vi "CCP_Main.vi"() -> ()   [LabVIEW 2019]
uses:
  LabJackU3/temperature_status_LabJackU3.ctl
panel:
  in  "open_IVC_OC200":bool caption="open_THCD_400"
  out "IVC_OC200_P2":dbl caption="IVC P2" format="%_3e"
  out "IVC_OC200_P1":dbl caption="IVC P1" format="%_3e"
  out "IVC_OC200_ST":u32(colorbox)
  out "HeatTape_ST":u32(colorbox)
  in  "open_Heat_Tape":bool caption="open_THCD_400"
  in  "audio_onoff":bool caption="Audio Alarm"
  in  "disp_magnet_level":bool
  in  "disp_shell_volume":bool
  in  "disp_magnet_space":bool
  out "MccHat_P":dbl caption="psig" format="%.2f"
  out "MccHat_ST":u32(colorbox)
  in  "open_MccHat":bool caption="open_THCD_400"
  out "LJT4_P_HR3":dbl caption="psi" format="%.1f"
  out "FM2":dbl
  out "msg_subsys":string
  in  "open_LJT4":bool caption="open_THCD_400"
  out "LJT4_T":dbl caption="°F" format="%.1f"
  out "LJT4_P":dbl caption="psi" format="%.1f"
  out "LJT4_ST":u32(colorbox)
  in  "open_GVB":bool caption="open_THCD_400"
  out "GVB_turn":dbl caption="turn" format="%.2f"
  out "GVB_ST":u32(colorbox)
  out "MRB_opening":dbl caption="%"
  in  "open_MRB":bool caption="open_THCD_400"
  out "MRB_ST":u32(colorbox)
  in  "Interval":i32=1000 caption="ms"
  out "time_update":timestamp caption="Last Update" format="%<%Y-%m-%d %H:%M:%S>T"
  out "MagPS_ST":u32(colorbox)
  out "ITM10_ST":u32(colorbox)
  out "RPLCW_ST":u32(colorbox)
  out "LJU3_TC_ST":u32(colorbox)
  out "LS218_02_ST":u32(colorbox)
  out "LS218_01_ST":u32(colorbox)
  out "MCCETC03_T7":dbl caption="F" format="%.1f"
  out "MCCETC03_T6":dbl caption="F" format="%.1f"
  out "MCCETC03_ST":u32(colorbox)
  out "MCCETC02_ST":u32(colorbox)
  out "MCCETC01_ST":u32(colorbox)
  out "TPG361_ST":u32(colorbox)
  out "BGA244_ST":u32(colorbox)
  out "THCD401_ST":u32(colorbox)
  out "MG_ST":u32(colorbox)
  out "FV_ST":u32(colorbox)
  out "MKS670_He3_ST":u32(colorbox)
  out "MKS670_100_ST":u32(colorbox)
  out "MKS670_1000_ST":u32(colorbox)
  in  "control_lock":bool caption="Control"
  in  "stop_all":bool caption="open_THCD_400"
  in  "start_all":bool caption="open_THCD_400"
  out "MKS946_ST":u32(colorbox)
  out "LS218_02_T8":dbl format="%.1f"
  out "level_fridge_LHe":dbl(slide) caption="%" scale=0.0..45.0 scale format="%#.1f"
  out "level_fridge_LN2":dbl(slide) caption="%" scale=0.0..100.0 scale format="%#.1f"
  out "MCCETC02_T7":dbl caption="Sep. Line" format="%.1f"
  in  "open_RPLCW":bool caption="open_THCD_400"
  out "RPLCW_WFS1":dbl caption="WFS1" format="%.1f"
  out "RPLCW_M4":dbl caption="M4" format="%.1f"
  out "RPLCW_M3":dbl caption="M3" format="%.1f"
  out "PRLCW_M2":dbl caption="M2" format="%.1f"
  out "RPLCW_M1":dbl caption="M1" format="%.1f"
  in  "open_LS218_02":bool caption="open_THCD_400"
  out "LS218_02_T7":dbl format="%.1f"
  out "LS218_02_T6":dbl format="%.1f"
  out "LS218_02_T5":dbl format="%.1f"
  out "LS218_02_T4":dbl format="%.1f"
  out "LS218_02_T3":dbl caption="W" format="%.1f"
  out "LS218_02_T2":dbl format="%.1f"
  out "LS218_02_T1":dbl caption="W" format="%.1f"
  out "Nose LHe Level":dbl(slide) caption="%" scale=0.0..100.0 scale format="%#_1f"
  in  "open_MagPS":bool caption="open_THCD_400"
  out "LS218_01_T8":dbl caption="W"
  out "LS218_01_T7":dbl caption="W"
  out "LS218_01_T6":dbl caption="W"
  out "LS218_01_T5":dbl caption="W"
  out "LS218_01_T4":dbl caption="W"
  out "LS218_01_T3":dbl caption="W"
  out "LS218_01_T2":dbl caption="W"
  out "LS218_01_T1":dbl caption="W"
  out "FC1":dbl
  out "FC2":dbl
  out "FM1":dbl
  in  "open_THCD_401":bool caption="open_THCD_400"
  out "MCCETC03_T5":dbl format="%.1f"
  out "MCCETC03_T4":dbl format="%.1f"
  in  "open_ITM10":bool caption="open_THCD_400"
  out "T_Coil_B":dbl caption="Coil B"
  out "T_Coil_T":dbl caption="Coil T"
  out "T_Tank_B":dbl caption="Tank B"
  out "T_Tank_T":dbl caption="Tank T"
  out "MG5":dbl caption="psi" format="%.1f"
  in  "open_LJU3_TC":bool caption="open_THCD_400"
  out "LJU3_T_status":T1=enum."UNKNOWN" caption="QT Comp. LCW Temp."
  out "p_mks670_100":dbl caption="Torr"
  in  "open_LS218_01":bool caption="open_THCD_400"
  in  "open_MCCETC03":bool caption="open_THCD_400"
  out "MCCETC03_T3":dbl caption="T3" format="%.1f"
  out "MCCETC03_T2":dbl caption="T2" format="%.1f"
  out "MCCETC03_T1":dbl caption="T1" format="%.1f"
  out "MCCETC03_T0":dbl caption="T0" format="%.1f"
  in  "open_MCCETC01":bool caption="open_THCD_400"
  out "MCCETC01_T7":dbl caption="DR" format="%.1f"
  out "MCCETC01_T6":dbl caption="DL" format="%.1f"
  out "MCCETC01_T5":dbl caption="DB" format="%.1f"
  out "MCCETC01_T4":dbl caption="DT" format="%.1f"
  out "MCCETC01_T3":dbl caption="UR" format="%.1f"
  out "MCCETC01_T2":dbl caption="UL" format="%.1f"
  out "MCCETC01_T1":dbl caption="UB" format="%.1f"
  out "MCCETC01_T0":dbl caption="UT" format="%.1f"
  out "MCCETC02_T6":dbl caption="Sep. Line" format="%.1f"
  out "MCCETC02_T5":dbl caption="LHe FL #2" format="%.1f"
  out "MCCETC02_T4":dbl caption="LHe FL #1" format="%.1f"
  out "MCCETC02_T3":dbl caption="LHe FL Stinger" format="%.1f"
  out "MCCETC02_T2":dbl caption="Fridge Top" format="%.1f"
  in  "open_MCCETC02":bool caption="open_THCD_400"
  out "MCCETC02_T1":dbl caption="IVC Top" format="%.2f"
  out "MCCETC02_T0":dbl caption="IVC Bottom" format="%.2f"
  in  "open_TPG361":bool caption="open_THCD_400"
  out "TPG361_p":dbl caption="IVC" format="%_3e"
  in  "open_BGA244":bool caption="open_THCD_400"
  out "Purity":dbl caption="%" format="%.2f"
  in  "stop":bool
  in  "open_MaxiGauge":bool
  out "MG4":dbl format="%_4f"
  out "MG3":dbl format="%_4f"
  out "MG2":dbl caption="Torr" format="%_4f"
  out "MG1":dbl caption="Torr" format="%_4f"
  in  "open_Fridge_Valve":bool
  in  "open_MKS670_He3":bool
  in  "open_MKS670_100":bool
  in  "open_MKS670_1000":bool
  out "Bypass Valve":dbl format="%_3f"
  out "P2":dbl caption="Root Exhaust" format="%.2f"
  out "He3 Vapor Pressure":dbl
  out "p_mks670_1000":dbl caption="Torr"
  out "Run-Valve":dbl format="%_3f"
  out "P1":dbl caption="QT Manifold" format="%.2f"
  in  "open_MKS946":bool
  # "Expert Control"
  # "Cryo Control Panel"
  # "Fridge Temperatures"
  # "GPM"
  # "Torr"
  # "Click a reading and stay for 1 sec to find its controller name."
  # "psi"
  # "Controller"
  # "Status"
  # "Sub Panel"
  # "MKS 670 / 1000"
  # "Fridge pressure upto 1000 Torr."
  # "Microwave System"
  # "L/m"
  # "EIO Tube"
  # "EIO Top"
  # "MKS 670 /   100"
  # "Fridge pressure upto 100 Torr."
  # "psi"
  # "°C"
  # "MKS 670 / He3"
  # "Fridge pressure with He3 probe."
  # "MKS 946"
  # "Return line pressures."
  # "THCD-401"
  # "Return flow control/monitor."
  # "Turns"
  # "MaxiGauge"
  # "Return line pressures."
  # "L/m"
  # "L/m"
  # "Outside gHe Tank"
  # "°C"
  # "°C"
  # "Fridge Valve"
  # "Fridge valves.  LHe level."
  # "Auto"
  # "Torr"
  # "Torr"
  # "BGA244"
  # "Helium purity."
  # "°C"
  # "HR3"
  # "TPG361"
  # "IVC pressure."
  # "L/m"
  # "ITM10"
  # "Magnet temperatures."
  # "Turns"
  # "MCC E-TC #01"
  # "Magnet pipe temperatures."
  # "MCC E-TC #02"
  # "Surface temperatures."
  # "K"
  # "MCC E-TC #03"
  # "Annealing, microwave, and heat-tape temp."
  # "°C"
  # "K"
  # "Target-Cup\nTemperatures"
  # "LakeShore218 #01"
  # "Fridge temperatures."
  # "°C"
  # "°C"
  # "LakeShore218 #02"
  # "Target temperatures."
  # "Roots-Pump LCW"
  # "Roots-pump LCW flows."
  # "K"
  # "°C"
  # "K"
  # "LabJack U3"
  # "Compressor LCW temperatures."
  # "Torr"
  # "LabJack T4"
  # "Outside gHe tank."
  # "K"
  # "Magnet PS"
  # "Magnet current.  LHe & LN2 levels."
  # "W"
  # "°C"
  # "%"
  # "MR Bypass"
  # "Magnet return bypass valve."
  # "Auto"
  # "K"
  # "GV Bypass"
  # "Gate-valve bypass valve."
  # "Auto"
  # "K"
  # "MCC HAT #01"
  # "Magnet pressure."
  # "Magnet Surface Temperature"
  # "%"
  # "°C"
  # "Heat Tape"
  # "IVC & Turret heat tape."
  # "K"
  # "IVC Turbo Pressure"
  # "IVC_OC200"
  # "Schematic Version 8.0"
  # "K"
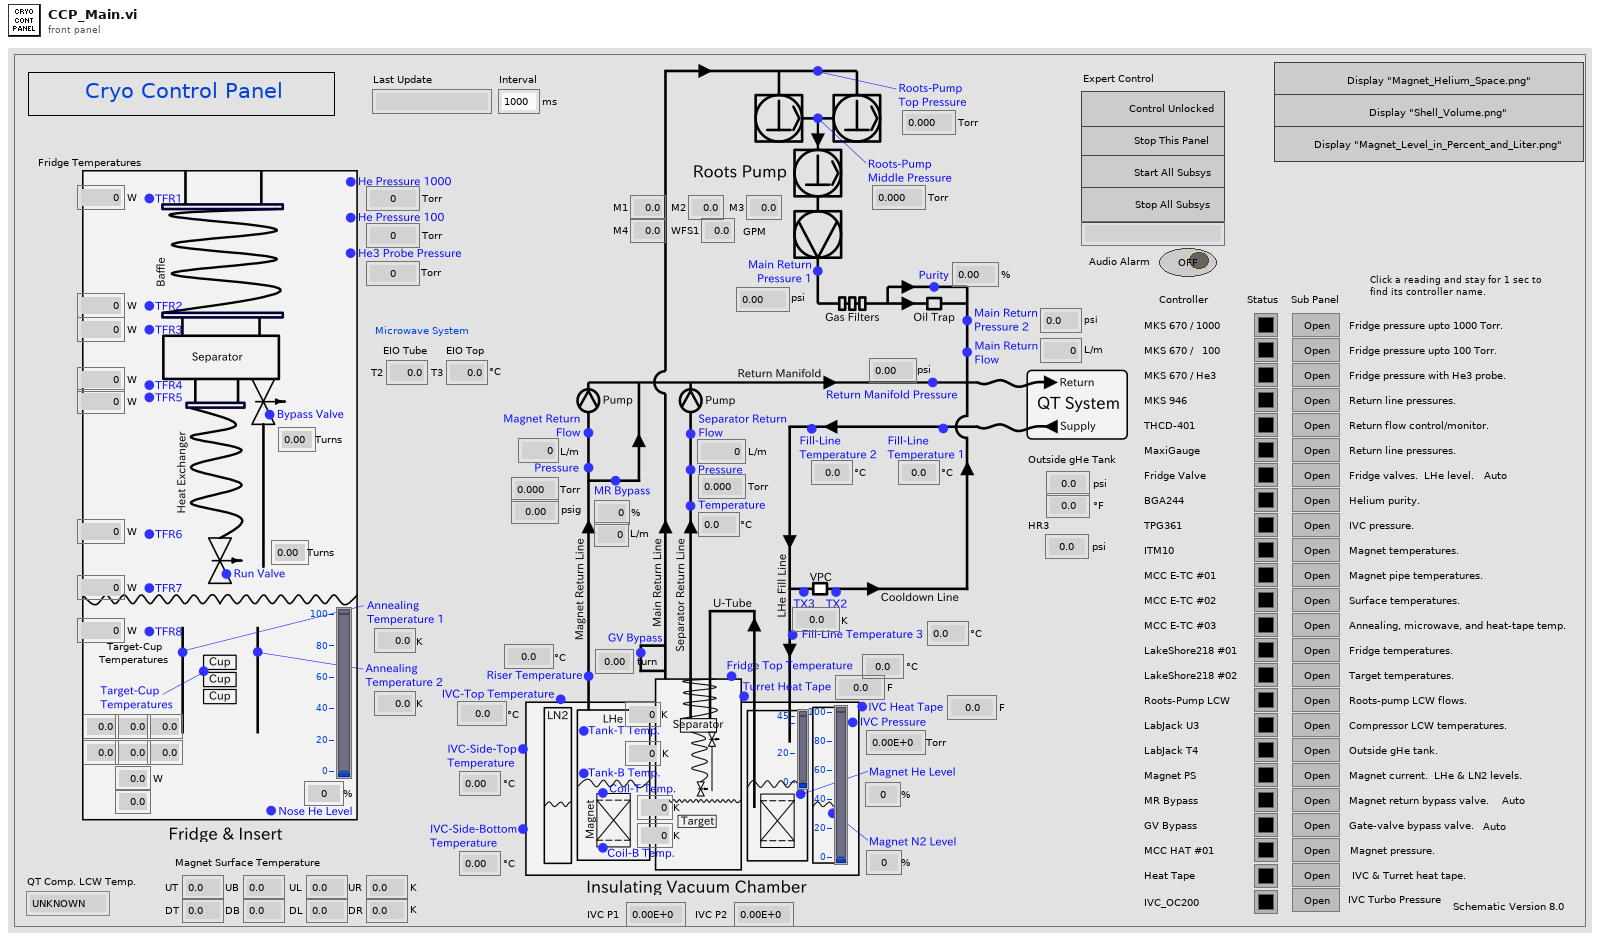
[diagram p1: front panel]
types:
  T1 = typedef "temperature_status_LabJackU3.ctl" = enum16{"OK", "UNKNOWN", "WARNING", "ERROR"}
  T2 = enum8{"Enabled", "Disabled", "Disabled and Grayed Out"}
  T3 = enum32{"Bad", "Idle", "Run top level", "Running"}
  T4 = cluster{"ITM10_ST":u32, "ITM10_Tank_T":dbl, "ITM10_Tank_B":dbl, "ITM10_Coil_T":dbl, "ITM10_Coil_B":dbl}
  T5 = cluster{"THCD401_ST":u32, "THCD401_FC1":dbl, "THCD401_FC2":dbl, "THCD401_FM1":dbl, "THCD401_FM2":dbl}
  T6 = cluster{"FV_ST":u32, "FV_run_valve":dbl, "FV_bypass_valve":dbl, "FV_nose_level":dbl}
  T7 = cluster{"MG_ST":u32, "MG_P1":dbl, "MG_P2":dbl, "MG_P3":dbl, "MG_P4":dbl, "MG_P5":dbl}
  T8 = cluster{"MKS670_1000_ST":u32, "MKS670_1000_P":dbl, "MKS670_1000_ST":u32, "MKS670_100_P":dbl, "MKS670_1000_ST":u32, "MKS670_He3_P":dbl}
  T9 = cluster{"MKS670_1000_ST":u32, "MKS946_P1":dbl, "MKS946_P2":dbl}
  T10 = cluster{"RPLCW_ST":u32, "RPLCW_M1":dbl, "RPLCW_M2":dbl, "RPLCW_M3":dbl, "RPLCW_M4":dbl, "RPLCW_WFS1":dbl}
  T11 = cluster{"LS218_02_ST":u32, "LS218_02_T1":dbl, "LS218_02_T2":dbl, "LS218_02_T3":dbl, "LS218_02_T4":dbl, "LS218_02_T5":dbl, "LS218_02_T6":dbl, "LS218_02_T7":dbl, "LS218_02_T8":dbl}
  T12 = cluster{"LS218_01_ST":u32, "LS218_01_T1":dbl, "LS218_01_T2":dbl, "LS218_01_T3":dbl, "LS218_01_T4":dbl, "LS218_01_T5":dbl, "LS218_01_T6":dbl, "LS218_01_T7":dbl, "LS218_01_T8":dbl}
  T13 = cluster{"MCCETC03_ST":u32, "MCCETC03_T0":dbl, "MCCETC03_T1":dbl, "MCCETC03_T2":dbl, "MCCETC03_T3":dbl, "MCCETC03_T4":dbl, "MCCETC03_T5":dbl, "MCCETC03_T6":dbl, "MCCETC03_T7":dbl}
  T14 = cluster{"MCCETC02_ST":u32, "MCCETC02_T0":dbl, "MCCETC02_T1":dbl, "MCCETC02_T2":dbl, "MCCETC02_T3":dbl, "MCCETC02_T4":dbl, "MCCETC02_T5":dbl, "MCCETC02_T6":dbl, "MCCETC02_T7":dbl}
  T15 = cluster{"MCCETC01_ST":u32, "MCCETC01_T0":dbl, "MCCETC01_T1":dbl, "MCCETC01_T2":dbl, "MCCETC01_T3":dbl, "MCCETC01_T4":dbl, "MCCETC01_T5":dbl, "MCCETC01_T6":dbl, "MCCETC01_T7":dbl}
  T16 = cluster{"LJT4_ST":u32, "LJT4_P":dbl, "LJT4_T":dbl, "LJT4_P_HR3":dbl}
  T17 = cluster{"MagPS_ST":u32, "MagPS_LHe":dbl, "MagPS_LN2":dbl}
  T18 = cluster{"HeatTape_ST":u32, "HeatTape_T1":dbl, "HeatTape_T2":dbl}
  T19 = cluster{"IVC_OC200_ST":u32, "IVC_OC200_P1":dbl, "IVC_OC200_P2":dbl}
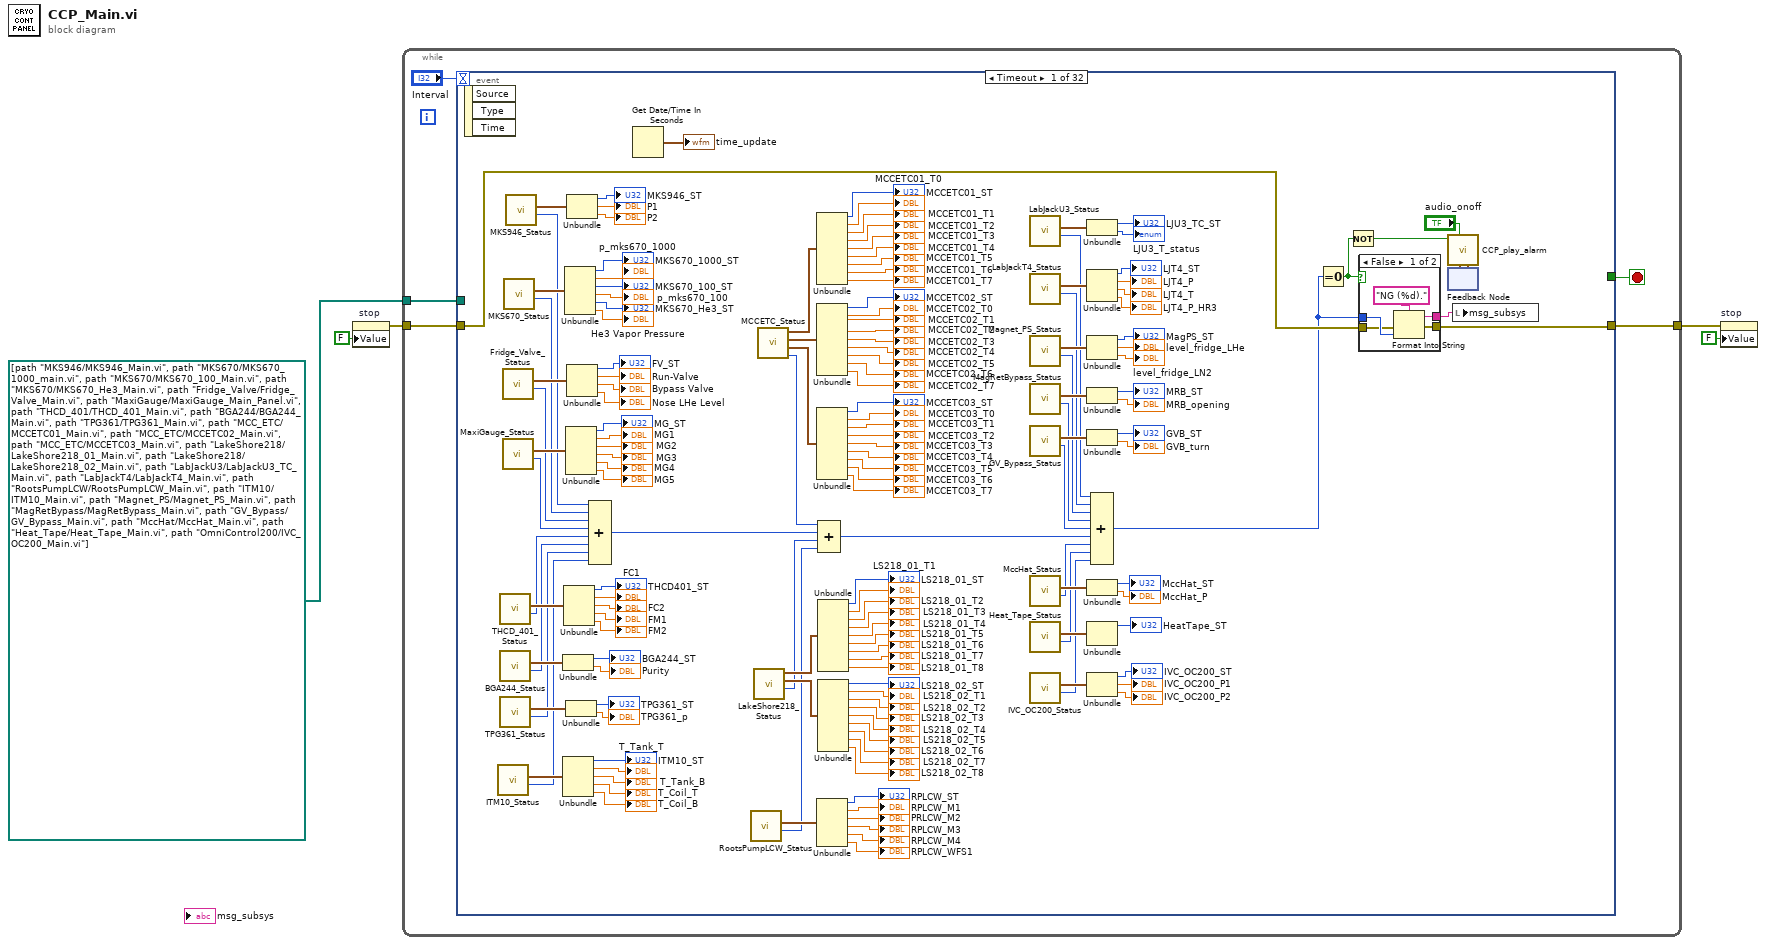
[diagram p0: block diagram]
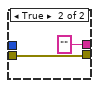
[diagram p2: hidden frame]
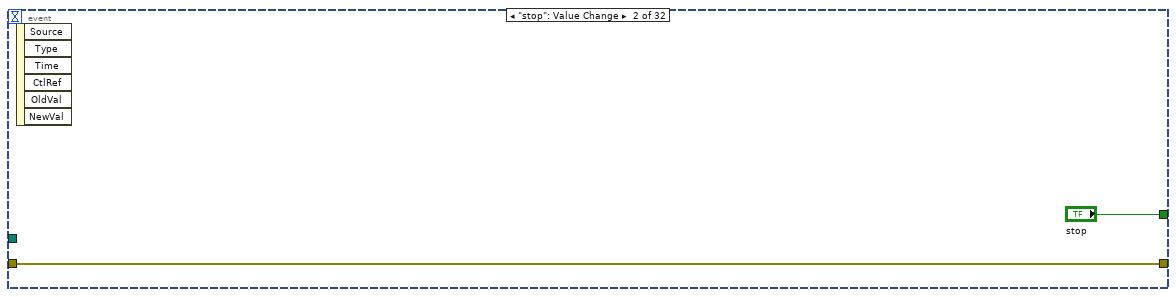
[diagram p3: hidden frame]
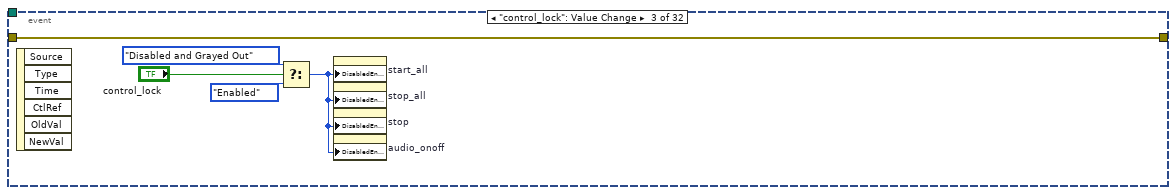
[diagram p4: hidden frame]
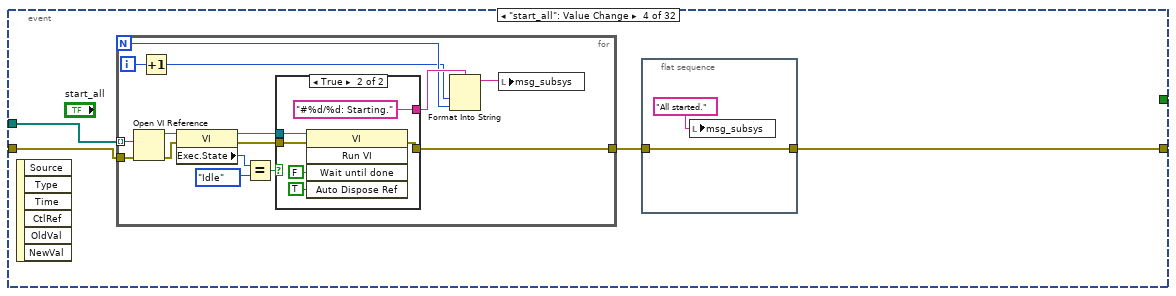
[diagram p5: hidden frame]
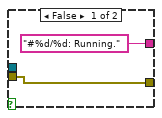
[diagram p6: hidden frame]
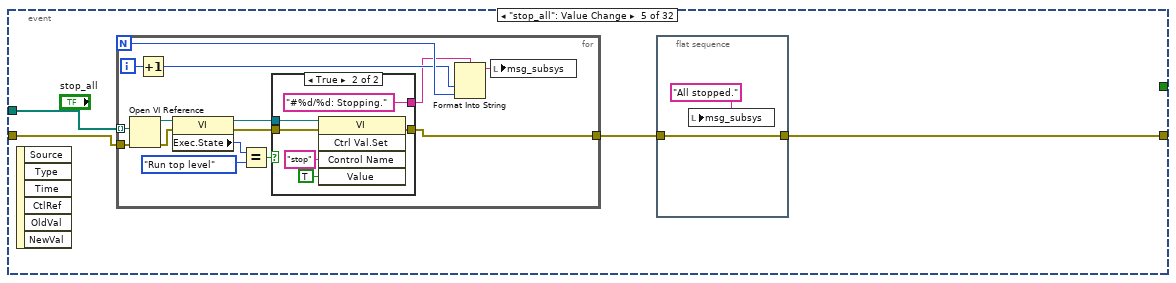
[diagram p7: hidden frame]
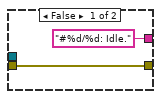
[diagram p8: hidden frame]
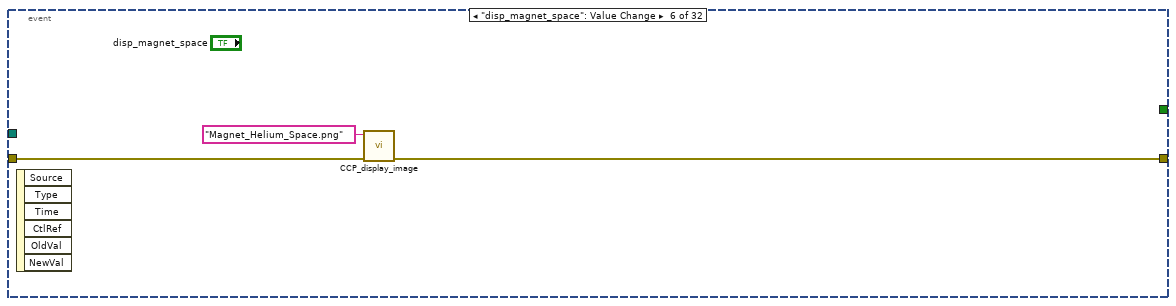
[diagram p9: hidden frame]
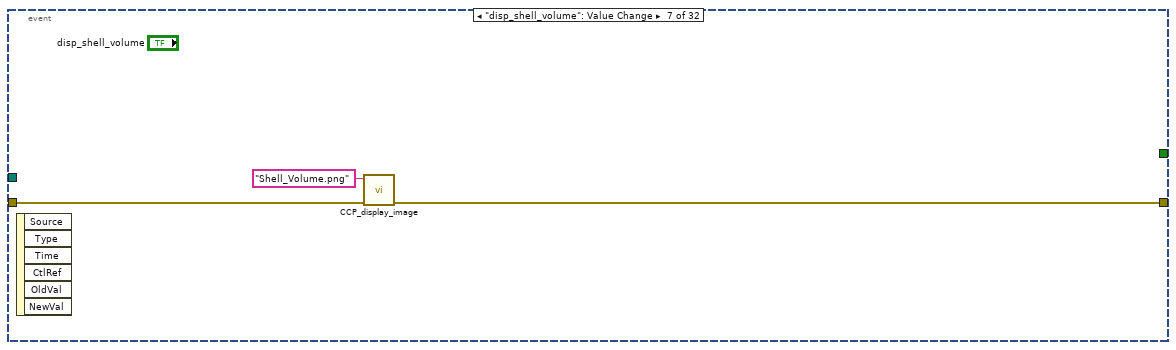
[diagram p10: hidden frame]
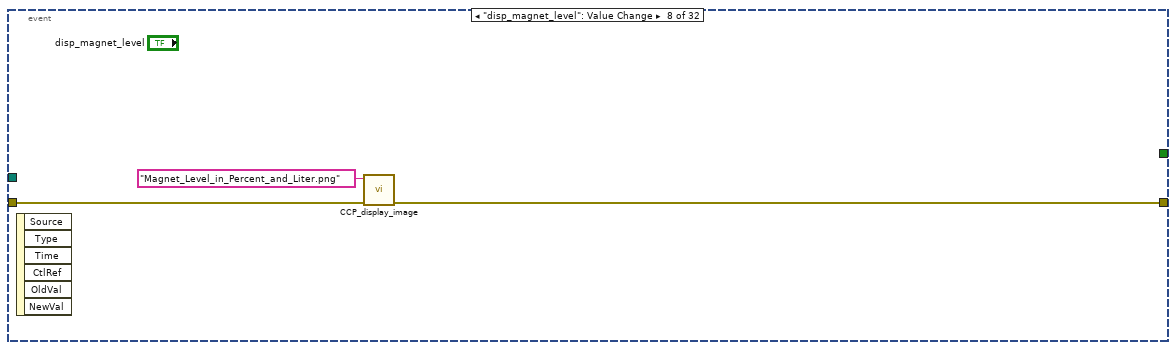
[diagram p11: hidden frame]
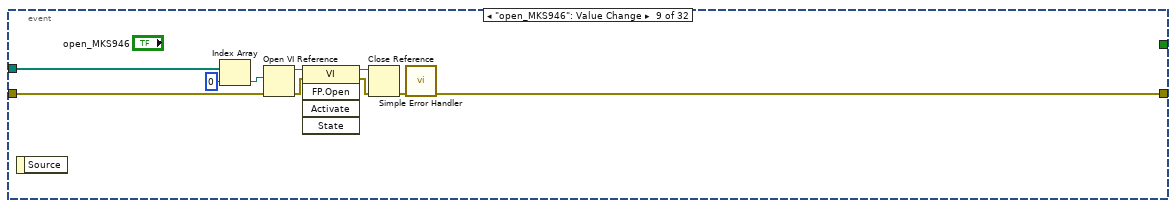
[diagram p12: hidden frame]
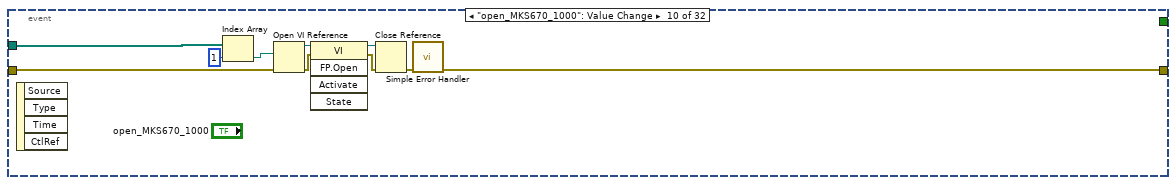
[diagram p13: hidden frame]
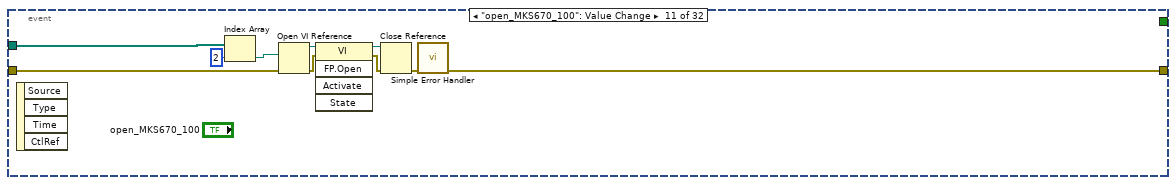
[diagram p14: hidden frame]
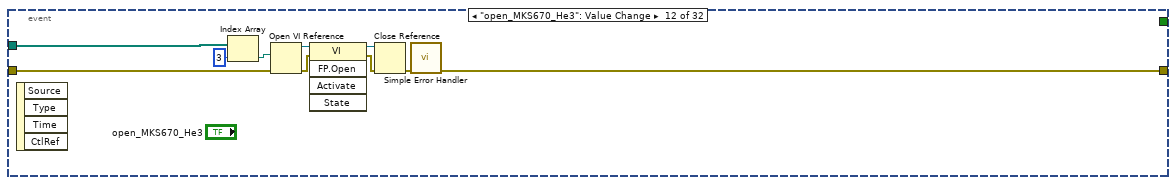
[diagram p15: hidden frame]
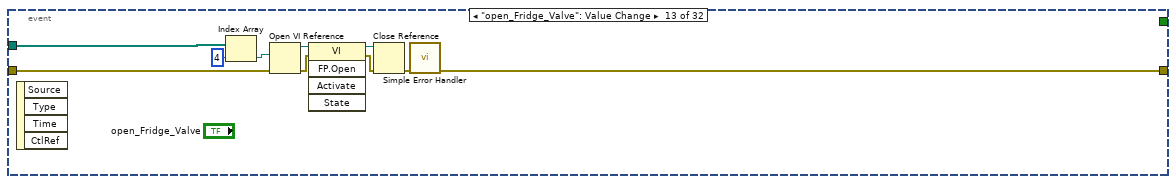
[diagram p16: hidden frame]
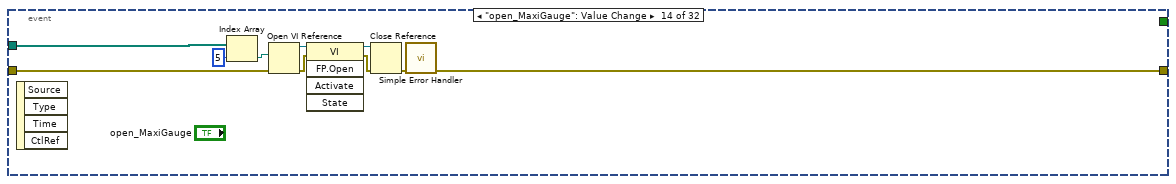
[diagram p17: hidden frame]
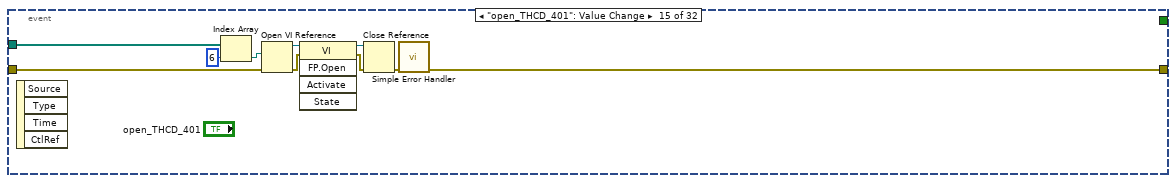
[diagram p18: hidden frame]
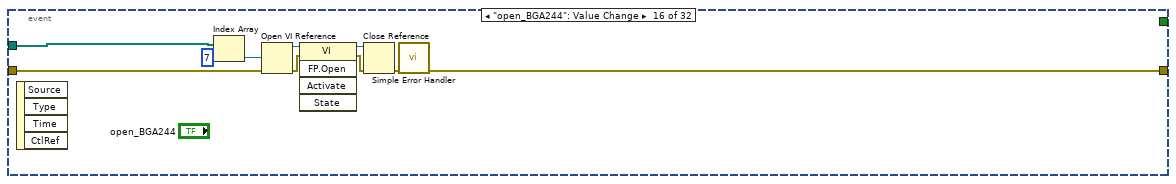
[diagram p19: hidden frame]
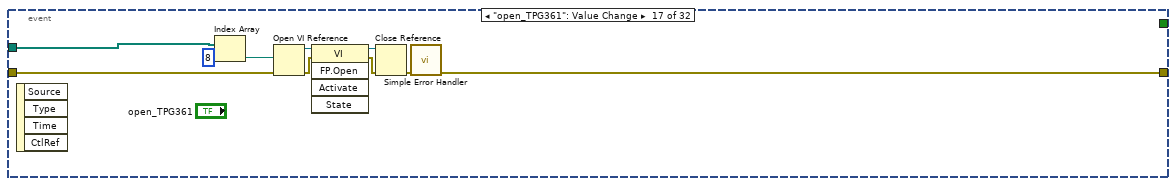
[diagram p20: hidden frame]
diagram:
  n1 = property on="stop" class="Bool (strict)"("Value"=FALSE ("all_stop_button")) -> (error out=w4:errorcluster)  [unwired: 2 in, 1 out]
  n2 = while {
    tunnel: w4 -> [w10]
    tunnel: [w7] -> w2
    tunnel: path[] [path "MKS946/MKS946_Main.vi", path "MKS670/MKS670_1000_main.vi", path "MKS670/MKS670_100_Main.vi", path "MKS670/MKS670_He3_Main.vi", path "Fridge_Valve/Fridge_Valve_Main.vi", path "MaxiGauge/MaxiGauge_Main_Panel.vi", path "THCD_401/THCD_401_Main.vi", path "BGA244/BGA244_Main.vi", path "TPG361/TPG361_Main.vi", path "MCC_ETC/MCCETC01_Main.vi", path "MCC_ETC/MCCETC02_Main.vi", path "MCC_ETC/MCCETC03_Main.vi", path "LakeShore218/LakeShore218_01_Main.vi", path "LakeShore218/LakeShore218_02_Main.vi", path "LabJackU3/LabJackU3_TC_Main.vi", path "LabJackT4/LabJackT4_Main.vi", path "RootsPumpLCW/RootsPumpLCW_Main.vi", path "ITM10/ITM10_Main.vi", path "Magnet_PS/Magnet_PS_Main.vi", path "MagRetBypass/MagRetBypass_Main.vi", path "GV_Bypass/GV_Bypass_Main.vi", path "MccHat/MccHat_Main.vi", path "Heat_Tape/Heat_Tape_Main.vi", path "OmniControl200/IVC_OC200_Main.vi"] -> [w9]
    stop <- w6 stop-if-true
    n3 = event shown="[0] Timeout" {
      selector: _ -> [_ _ _ _ _ _ _ _ _ _ _ _ _ _ _ _ _ _ _ _ _ _ _ _ _ _ _ _ _ _ _ _]
      dyn-events: _ -> [_ _ _ _ _ _ _ _ _ _ _ _ _ _ _ _ _ _ _ _ _ _ _ _ _ _ _ _ _ _ _ _]
      timeout: "Interval" -> [_ _ _ _ _ _ _ _ _ _ _ _ _ _ _ _ _ _ _ _ _ _ _ _ _ _ _ _ _ _ _ _]
      tunnel: w10 -> [w166 w174 w177 w183 w212 w241 w244 w247 w252 w262 w272 w281 w292 w302 w312 w322 w332 w342 w352 w362 w372 w382 w392 w402 w412 w422 w432 w442 w452 w462 w472 w482]
      tunnel: [w165 w174 w177 w181 w210 w240 w243 w246 w248 w261 w271 w280 w291 w301 w311 w321 w331 w341 w351 w361 w371 w381 w391 w401 w411 w421 w431 w441 w451 w461 w471 w481] -> w7
      tunnel: w9 -> [_ _ _ w184 w213 _ _ _ w249 w258 w268 w278 w289 w300 w308 w318 w328 w338 w349 w358 w369 w379 w389 w400 w409 w419 w429 w438 w449 w459 w469 w479]
      tunnel: [_ "stop" _ _ _ _ _ _ _ _ _ _ _ _ _ _ _ _ _ _ _ _ _ _ _ _ _ _ _ _ _ _] -> w6
      event Timeout {
        n4 = event-data() -> ()  [unwired: 1 in, 3 out]
        n5 = call "ITM10_Status.vi"() -> ("n_ng"=w25:u8, "values"=w82:T4)  [unwired: 10 in]
        n6 = call "THCD_401_Status.vi"() -> ("n_ng"=w28:u8, "values"=w145:T5)  [unwired: 10 in]
        n7 = call "BGA244_Status.vi"() -> ("n_ng"=w27:u8, "values"=w64:cluster{"BGA244_ST":u32, "BGA244_Purity":dbl})  [unwired: 10 in]
        n8 = call "TPG361_Status.vi"() -> ("n_ng"=w26:u8, "values"=w61:cluster{"TPG361_ST":u32, "TPG361_p":dbl})  [unwired: 10 in]
        n9 = call "Fridge_Valve_Status.vi"() -> ("n_ng"=w30:u8, "values"=w69:T6)  [unwired: 10 in]
        n10 = call "MaxiGauge_Status.vi"() -> ("n_ng"=w29:u8, "values"=w152:T7)  [unwired: 10 in]
        n11 = call "MKS670_Status.vi"() -> ("n_ng"=w31:u8, "values"=w163:T8)  [unwired: 10 in]
        n12 = call "MKS946_Status.vi"() -> ("n_ng"=w32:u8, "values"=w156:T9)  [unwired: 10 in]
        n13 = Unbundle(w64) -> ("BGA244_ST"=→"BGA244_ST":u32, "BGA244_Purity"=→"Purity":dbl)
        n14 = Unbundle(w82) -> ("ITM10_ST"=→"ITM10_ST":u32, "ITM10_Tank_T"=→"T_Tank_T":dbl, "ITM10_Tank_B"=→"T_Tank_B":dbl, "ITM10_Coil_T"=→"T_Coil_T":dbl, "ITM10_Coil_B"=→"T_Coil_B":dbl)
        n15 = Unbundle(w145) -> ("THCD401_ST"=→"THCD401_ST":u32, "THCD401_FC1"=→"FC1":dbl, "THCD401_FC2"=→"FC2":dbl, "THCD401_FM1"=→"FM1":dbl, "THCD401_FM2"=→"FM2":dbl)
        n16 = Unbundle(w163) -> ("MKS670_1000_ST"=→"MKS670_1000_ST":u32, "MKS670_1000_P"=→"p_mks670_1000":dbl, "MKS670_1000_ST"=→"MKS670_100_ST":u32, "MKS670_100_P"=→"p_mks670_100":dbl, "MKS670_1000_ST"=→"MKS670_He3_ST":u32, "MKS670_He3_P"=→"He3 Vapor Pressure":dbl)
        n17 = Unbundle(w152) -> ("MG_ST"=→"MG_ST":u32, "MG_P1"=→"MG1":dbl, "MG_P2"=→"MG2":dbl, "MG_P3"=→"MG3":dbl, "MG_P4"=→"MG4":dbl, "MG_P5"=→"MG5":dbl)
        n18 = Unbundle(w61) -> ("TPG361_ST"=→"TPG361_ST":u32, "TPG361_p"=→"TPG361_p":dbl)
        n19 = Unbundle(w156) -> ("MKS670_1000_ST"=→"MKS946_ST":u32, "MKS946_P1"=→"P1":dbl, "MKS946_P2"=→"P2":dbl)
        n20 = Unbundle(w69) -> ("FV_ST"=→"FV_ST":u32, "FV_run_valve"=→"Run-Valve":dbl, "FV_bypass_valve"=→"Bypass Valve":dbl, "FV_nose_level"=→"Nose LHe Level":dbl)
        n21 = Compound Arithmetic op=ADD(w32, w31, w30, w29, w28, w27, w26, w25) -> (w24:u8)
        n22 = Get Date/Time In Seconds() -> (seconds since 1Jan1904=→"time_update":timestamp)
        n23 = call "RootsPumpLCW_Status.vi"() -> ("n_ng"=w21:u8, "values"=w119:T10)  [unwired: 10 in]
        n24 = call "LakeShore218_Status.vi"() -> ("n_ng"=w22:u8, "value2"=w139:T11, "value1"=w138:T12)  [unwired: 9 in]
        n25 = call "MCCETC_Status.vi"() -> ("n_ng"=w23:u8, "values3"=w110:T13, "values2"=w111:T14, "values1"=w112:T15)  [unwired: 8 in]
        n26 = Unbundle(w112) -> ("MCCETC01_ST"=→"MCCETC01_ST":u32, "MCCETC01_T0"=→"MCCETC01_T0":dbl, "MCCETC01_T1"=→"MCCETC01_T1":dbl, "MCCETC01_T2"=→"MCCETC01_T2":dbl, "MCCETC01_T3"=→"MCCETC01_T3":dbl, "MCCETC01_T4"=→"MCCETC01_T4":dbl, "MCCETC01_T5"=→"MCCETC01_T5":dbl, "MCCETC01_T6"=→"MCCETC01_T6":dbl, "MCCETC01_T7"=→"MCCETC01_T7":dbl)
        n27 = Unbundle(w111) -> ("MCCETC02_ST"=→"MCCETC02_ST":u32, "MCCETC02_T0"=→"MCCETC02_T0":dbl, "MCCETC02_T1"=→"MCCETC02_T1":dbl, "MCCETC02_T2"=→"MCCETC02_T2":dbl, "MCCETC02_T3"=→"MCCETC02_T3":dbl, "MCCETC02_T4"=→"MCCETC02_T4":dbl, "MCCETC02_T5"=→"MCCETC02_T5":dbl, "MCCETC02_T6"=→"MCCETC02_T6":dbl, "MCCETC02_T7"=→"MCCETC02_T7":dbl)
        n28 = Unbundle(w110) -> ("MCCETC03_ST"=→"MCCETC03_ST":u32, "MCCETC03_T0"=→"MCCETC03_T0":dbl, "MCCETC03_T1"=→"MCCETC03_T1":dbl, "MCCETC03_T2"=→"MCCETC03_T2":dbl, "MCCETC03_T3"=→"MCCETC03_T3":dbl, "MCCETC03_T4"=→"MCCETC03_T4":dbl, "MCCETC03_T5"=→"MCCETC03_T5":dbl, "MCCETC03_T6"=→"MCCETC03_T6":dbl, "MCCETC03_T7"=→"MCCETC03_T7":dbl)
        n29 = Unbundle(w119) -> ("RPLCW_ST"=→"RPLCW_ST":u32, "RPLCW_M1"=→"RPLCW_M1":dbl, "RPLCW_M2"=→"PRLCW_M2":dbl, "RPLCW_M3"=→"RPLCW_M3":dbl, "RPLCW_M4"=→"RPLCW_M4":dbl, "RPLCW_WFS1"=→"RPLCW_WFS1":dbl)
        n30 = Compound Arithmetic op=ADD(w23, w24, w22, w21) -> (w15:u8)
        n31 = Unbundle(w138) -> ("LS218_01_ST"=→"LS218_01_ST":u32, "LS218_01_T1"=→"LS218_01_T1":dbl, "LS218_01_T2"=→"LS218_01_T2":dbl, "LS218_01_T3"=→"LS218_01_T3":dbl, "LS218_01_T4"=→"LS218_01_T4":dbl, "LS218_01_T5"=→"LS218_01_T5":dbl, "LS218_01_T6"=→"LS218_01_T6":dbl, "LS218_01_T7"=→"LS218_01_T7":dbl, "LS218_01_T8"=→"LS218_01_T8":dbl)
        n32 = Unbundle(w139) -> ("LS218_02_ST"=→"LS218_02_ST":u32, "LS218_02_T1"=→"LS218_02_T1":dbl, "LS218_02_T2"=→"LS218_02_T2":dbl, "LS218_02_T3"=→"LS218_02_T3":dbl, "LS218_02_T4"=→"LS218_02_T4":dbl, "LS218_02_T5"=→"LS218_02_T5":dbl, "LS218_02_T6"=→"LS218_02_T6":dbl, "LS218_02_T7"=→"LS218_02_T7":dbl, "LS218_02_T8"=→"LS218_02_T8":dbl)
        n33 = call "LabJackU3_Status.vi"() -> ("n_ng"=w20:u8, "values"=w72:cluster{"LJU3_ST":u32, "LJU3_TEMP_ST":T1})  [unwired: 10 in]
        n34 = call "LabJackT4_Status.vi"() -> ("n_ng"=w19:u8, "values"=w49:T16)  [unwired: 10 in]
        n35 = call "Magnet_PS_Status.vi"() -> ("n_ng"=w18:u8, "values"=w76:T17)  [unwired: 10 in]
        n36 = call "MagRetBypass_Status.vi"() -> ("n_ng"=w17:u8, "values"=w58:cluster{"MRB_ST":u32, "MRB_opening":dbl})  [unwired: 10 in]
        n37 = call "GV_Bypass_Status.vi"() -> ("n_ng"=w16:u8, "values"=w55:cluster{"GVB_ST":u32, "GVB_turn":dbl})  [unwired: 10 in]
        n38 = call "MccHat_Status.vi"() -> ("n_ng"=w14:u8, "values"=w52:cluster{"MccHat_ST":u32, "MccHat_P":dbl})  [unwired: 10 in]
        n39 = call "Heat_Tape_Status.vi"() -> ("n_ng"=w13:u8, "values"=w44:T18)  [unwired: 10 in]
        n40 = call "IVC_OC200_Status.vi"() -> ("n_ng"=w12:u8, "values"=w42:T19)  [unwired: 10 in]
        n41 = Unbundle(w72) -> ("LJU3_ST"=→"LJU3_TC_ST":u32, "LJU3_TEMP_ST"=→"LJU3_T_status":T1)
        n42 = Unbundle(w49) -> ("LJT4_ST"=→"LJT4_ST":u32, "LJT4_P"=→"LJT4_P":dbl, "LJT4_T"=→"LJT4_T":dbl, "LJT4_P_HR3"=→"LJT4_P_HR3":dbl)
        n43 = Unbundle(w76) -> ("MagPS_ST"=→"MagPS_ST":u32, "MagPS_LHe"=→"level_fridge_LHe":dbl, "MagPS_LN2"=→"level_fridge_LN2":dbl)
        n44 = Unbundle(w58) -> ("MRB_ST"=→"MRB_ST":u32, "MRB_opening"=→"MRB_opening":dbl)
        n45 = Unbundle(w55) -> ("GVB_ST"=→"GVB_ST":u32, "GVB_turn"=→"GVB_turn":dbl)
        n46 = Unbundle(w52) -> ("MccHat_ST"=→"MccHat_ST":u32, "MccHat_P"=→"MccHat_P":dbl)
        n47 = Unbundle(w44) -> ("HeatTape_ST"=→"HeatTape_ST":u32)  [unwired: 2 out]
        n48 = Unbundle(w42) -> ("IVC_OC200_ST"=→"IVC_OC200_ST":u32, "IVC_OC200_P1"=→"IVC_OC200_P1":dbl, "IVC_OC200_P2"=→"IVC_OC200_P2":dbl)
        n49 = Compound Arithmetic op=ADD(w20, w19, w18, w17, w16, w15, w14, w13, w12) -> (w11:u8)
        n50 = Equal To 0?(x=w11) -> (x = 0?=w38:bool)
        n51 = Not(x=w38) -> (.not. x?=w37:bool)
        n52 = case shown="False" w38 {
          tunnel: [w171 "" ("msg_subsys")] -> w34
          tunnel: w11 -> [w169 _]
          tunnel: w166 -> [w168 w172]
          tunnel: [w167 w172] -> w165
          frame False {
            n53 = Format Into String(format string="NG (%d).", error in=w168, w169) -> (resulting string=w171:string, error out=w167:errorcluster)  [unwired: 1 in]
          }
          frame True {
          }
        }
        n54 = feedback #1() -> (w36:timestamp[])  [unwired: 1 in]
        n55 = call "CCP_play_alarm.vi"("time_last_in"=w36, "audio_onoff"="audio_onoff", "error"=w37) -> ("time_last_out"=w33:timestamp[])  [unwired: 8 in]
        n56 = feedback-in #1(w33) -> ()
        n57 = local write "msg_subsys"(w34) -> ()
      }
      event "stop": Value Change {
        n58 = event-data() -> ()  [unwired: 1 in, 6 out]
      }
      event "control_lock": Value Change {
        n59 = event-data() -> ()  [unwired: 1 in, 6 out]
        n60 = Select(t=T2."Disabled and Grayed Out" ("Disabled"), s="control_lock", f=T2."Enabled" ("Disabled")) -> (s? t:f=w176:T2)
        n61 = property on="start_all" class="Bool"("DisabledEnum"=w176) -> ()  [unwired: 2 in, 2 out]
        n62 = property on="stop_all" class="Bool"("DisabledEnum"=w176) -> ()  [unwired: 2 in, 2 out]
        n63 = property on="stop" class="Bool (strict)"("DisabledEnum"=w176) -> ()  [unwired: 2 in, 2 out]
        n64 = property on="audio_onoff" class="Bool (strict)"("DisabledEnum"=w176) -> ()  [unwired: 2 in, 2 out]
      }
      event "start_all": Value Change {
        n65 = event-data() -> ()  [unwired: 1 in, 6 out]
        n66 = for {
          N -> [w188]
          tunnel: w184 -> [w194] mode=indexing
          tunnel: w183 -> [w193]
          tunnel: [w192] -> w182
          i -> [w190]
          n67 = Open VI Reference(vi path=w194, error in (no error)=w193) -> (vi reference=w201:refnum<vi>, error out=w200:errorcluster)  [unwired: 4 in]
          n68 = Increment(x=w190) -> (x+1=w187:i32)
          n69 = property class="VI"(reference=w201, error in=w200) -> (reference out=w199:refnum<vi>, error out=w198:errorcluster, "Exec.State"=w197:T3)
          n70 = Equal?(x=w197, y=T3."Idle" ("Execution:State")) -> (x = y?=w195:bool)
          n71 = case shown="True" w195 {
            tunnel: w199 -> [_ w207]
            tunnel: w198 -> [w203 w206]
            tunnel: [w203 w205] -> w192
            tunnel: ["#%d/%d: Running." ("format string") "#%d/%d: Starting." ("format string")] -> w189
            frame False {
            }
            frame True {
              n72 = invoke class="VI" method="Run VI"(reference=w207, error in=w206, "Wait until done"=FALSE ("Wait Until Done"), "Auto Dispose Ref"=TRUE ("Auto Dispose Reference")) -> (error out=w205:errorcluster)  [unwired: 1 in, 4 out]
            }
          }
          n73 = Format Into String(format string=w189, w187, w188) -> (resulting string=w191:string)  [unwired: 2 in, 1 out]
          n74 = local write "msg_subsys"(w191) -> ()
        }
        n75 = flat-sequence {
          tunnel: w182 -> [w186]
          tunnel: [w186] -> w181
          frame #0 {
            n76 = local write "msg_subsys"("All started." ("msg_subsys")) -> ()
          }
        }
      }
      event "stop_all": Value Change {
        n77 = event-data() -> ()  [unwired: 1 in, 6 out]
        n78 = for {
          N -> [w218]
          tunnel: w213 -> [w223] mode=indexing
          tunnel: w212 -> [w222]
          tunnel: [w221] -> w211
          i -> [w219]
          n79 = Open VI Reference(vi path=w223, error in (no error)=w222) -> (vi reference=w230:refnum<vi>, error out=w229:errorcluster)  [unwired: 4 in]
          n80 = Increment(x=w219) -> (x+1=w217:i32)
          n81 = property class="VI"(reference=w230, error in=w229) -> (reference out=w228:refnum<vi>, error out=w227:errorcluster, "Exec.State"=w226:T3)
          n82 = Equal?(x=w226, y=T3."Run top level" ("Execution:State")) -> (x = y?=w224:bool)
          n83 = case shown="True" w224 {
            tunnel: w228 -> [_ w237]
            tunnel: w227 -> [w232 w236]
            tunnel: [w232 w234] -> w221
            tunnel: ["#%d/%d: Idle." ("format string") "#%d/%d: Stopping." ("format string")] -> w216
            frame False {
            }
            frame True {
              n84 = invoke class="VI" method="Ctrl Val.Set"(reference=w237, error in=w236, "Control Name"="stop", "Value"=TRUE ("Auto Dispose Reference")) -> (error out=w234:errorcluster)  [unwired: 1 in, 4 out]
            }
          }
          n85 = Format Into String(format string=w216, w217, w218) -> (resulting string=w220:string)  [unwired: 2 in, 1 out]
          n86 = local write "msg_subsys"(w220) -> ()
        }
        n87 = flat-sequence {
          tunnel: w211 -> [w215]
          tunnel: [w215] -> w210
          frame #0 {
            n88 = local write "msg_subsys"("All stopped." ("msg_subsys")) -> ()
          }
        }
      }
      event "disp_magnet_space": Value Change {
        n89 = event-data() -> ()  [unwired: 1 in, 6 out]
        n90 = call "CCP_display_image.vi"("error in"=w241, "file_name"="Magnet_Helium_Space.png") -> ("error out"=w240:errorcluster)  [unwired: 7 in, 2 out]
      }
      event "disp_shell_volume": Value Change {
        n91 = event-data() -> ()  [unwired: 1 in, 6 out]
        n92 = call "CCP_display_image.vi"("error in"=w244, "file_name"="Shell_Volume.png") -> ("error out"=w243:errorcluster)  [unwired: 7 in, 2 out]
      }
      event "disp_magnet_level": Value Change {
        n93 = event-data() -> ()  [unwired: 1 in, 6 out]
        n94 = call "CCP_display_image.vi"("error in"=w247, "file_name"="Magnet_Level_in_Percent_and_Liter.png") -> ("error out"=w246:errorcluster)  [unwired: 7 in, 2 out]
      }
      event "open_MKS946": Value Change {
        n95 = event-data() -> ()  [unwired: 1 in, 1 out]
        n96 = Index Array(array=w249, index=0) -> (element=w250:path)
        n97 = Open VI Reference(vi path=w250, error in (no error)=w252) -> (vi reference=w253:refnum<vi>, error out=w254:errorcluster)  [unwired: 4 in]
        n98 = invoke class="VI" method="FP.Open"(reference=w253, error in=w254) -> (reference out=w256:refnum<vi>, error out=w257:errorcluster)  [unwired: 3 in, 3 out]
        n99 = Close Reference(reference=w256, error in (no error)=w257) -> (error out=w255:errorcluster)
        n100 = call <vilib>:"Simple Error Handler.vi"("error in (no error)"=w255) -> ("error out"=w248:errorcluster)  [unwired: 4 in, 4 out]
      }
      event "open_MKS670_1000": Value Change {
        n101 = event-data() -> ()  [unwired: 1 in, 4 out]
        n102 = Index Array(array=w258, index=1) -> (element=w259:path)
        n103 = Open VI Reference(vi path=w259, error in (no error)=w262) -> (vi reference=w263:refnum<vi>, error out=w264:errorcluster)  [unwired: 4 in]
        n104 = invoke class="VI" method="FP.Open"(reference=w263, error in=w264) -> (reference out=w266:refnum<vi>, error out=w267:errorcluster)  [unwired: 3 in, 3 out]
        n105 = Close Reference(reference=w266, error in (no error)=w267) -> (error out=w265:errorcluster)
        n106 = call <vilib>:"Simple Error Handler.vi"("error in (no error)"=w265) -> ("error out"=w261:errorcluster)  [unwired: 4 in, 4 out]
      }
      event "open_MKS670_100": Value Change {
        n107 = event-data() -> ()  [unwired: 1 in, 4 out]
        n108 = Index Array(array=w268, index=2) -> (element=w269:path)
        n109 = Open VI Reference(vi path=w269, error in (no error)=w272) -> (vi reference=w277:refnum<vi>, error out=w276:errorcluster)  [unwired: 4 in]
        n110 = invoke class="VI" method="FP.Open"(reference=w277, error in=w276) -> (reference out=w274:refnum<vi>, error out=w273:errorcluster)  [unwired: 3 in, 3 out]
        n111 = Close Reference(reference=w274, error in (no error)=w273) -> (error out=w275:errorcluster)
        n112 = call <vilib>:"Simple Error Handler.vi"("error in (no error)"=w275) -> ("error out"=w271:errorcluster)  [unwired: 4 in, 4 out]
      }
      event "open_MKS670_He3": Value Change {
        n113 = event-data() -> ()  [unwired: 1 in, 4 out]
        n114 = Index Array(array=w278, index=3) -> (element=w279:path)
        n115 = Open VI Reference(vi path=w279, error in (no error)=w281) -> (vi reference=w287:refnum<vi>, error out=w286:errorcluster)  [unwired: 4 in]
        n116 = invoke class="VI" method="FP.Open"(reference=w287, error in=w286) -> (reference out=w284:refnum<vi>, error out=w283:errorcluster)  [unwired: 3 in, 3 out]
        n117 = Close Reference(reference=w284, error in (no error)=w283) -> (error out=w285:errorcluster)
        n118 = call <vilib>:"Simple Error Handler.vi"("error in (no error)"=w285) -> ("error out"=w280:errorcluster)  [unwired: 4 in, 4 out]
      }
      event "open_Fridge_Valve": Value Change {
        n119 = event-data() -> ()  [unwired: 1 in, 4 out]
        n120 = Index Array(array=w289, index=4) -> (element=w290:path)
        n121 = Open VI Reference(vi path=w290, error in (no error)=w292) -> (vi reference=w297:refnum<vi>, error out=w296:errorcluster)  [unwired: 4 in]
        n122 = invoke class="VI" method="FP.Open"(reference=w297, error in=w296) -> (reference out=w294:refnum<vi>, error out=w293:errorcluster)  [unwired: 3 in, 3 out]
        n123 = Close Reference(reference=w294, error in (no error)=w293) -> (error out=w295:errorcluster)
        n124 = call <vilib>:"Simple Error Handler.vi"("error in (no error)"=w295) -> ("error out"=w291:errorcluster)  [unwired: 4 in, 4 out]
      }
      event "open_MaxiGauge": Value Change {
        n125 = event-data() -> ()  [unwired: 1 in, 4 out]
        n126 = Index Array(array=w300, index=5) -> (element=w299:path)
        n127 = Open VI Reference(vi path=w299, error in (no error)=w302) -> (vi reference=w307:refnum<vi>, error out=w306:errorcluster)  [unwired: 4 in]
        n128 = invoke class="VI" method="FP.Open"(reference=w307, error in=w306) -> (reference out=w304:refnum<vi>, error out=w303:errorcluster)  [unwired: 3 in, 3 out]
        n129 = Close Reference(reference=w304, error in (no error)=w303) -> (error out=w305:errorcluster)
        n130 = call <vilib>:"Simple Error Handler.vi"("error in (no error)"=w305) -> ("error out"=w301:errorcluster)  [unwired: 4 in, 4 out]
      }
      event "open_THCD_401": Value Change {
        n131 = event-data() -> ()  [unwired: 1 in, 4 out]
        n132 = Index Array(array=w308, index=6) -> (element=w309:path)
        n133 = Open VI Reference(vi path=w309, error in (no error)=w312) -> (vi reference=w313:refnum<vi>, error out=w314:errorcluster)  [unwired: 4 in]
        n134 = invoke class="VI" method="FP.Open"(reference=w313, error in=w314) -> (reference out=w316:refnum<vi>, error out=w317:errorcluster)  [unwired: 3 in, 3 out]
        n135 = Close Reference(reference=w316, error in (no error)=w317) -> (error out=w315:errorcluster)
        n136 = call <vilib>:"Simple Error Handler.vi"("error in (no error)"=w315) -> ("error out"=w311:errorcluster)  [unwired: 4 in, 4 out]
      }
      event "open_BGA244": Value Change {
        n137 = event-data() -> ()  [unwired: 1 in, 4 out]
        n138 = Index Array(array=w318, index=7) -> (element=w319:path)
        n139 = Open VI Reference(vi path=w319, error in (no error)=w322) -> (vi reference=w323:refnum<vi>, error out=w324:errorcluster)  [unwired: 4 in]
        n140 = invoke class="VI" method="FP.Open"(reference=w323, error in=w324) -> (reference out=w326:refnum<vi>, error out=w327:errorcluster)  [unwired: 3 in, 3 out]
        n141 = Close Reference(reference=w326, error in (no error)=w327) -> (error out=w325:errorcluster)
        n142 = call <vilib>:"Simple Error Handler.vi"("error in (no error)"=w325) -> ("error out"=w321:errorcluster)  [unwired: 4 in, 4 out]
      }
      event "open_TPG361": Value Change {
        n143 = event-data() -> ()  [unwired: 1 in, 4 out]
        n144 = Index Array(array=w328, index=8) -> (element=w329:path)
        n145 = Open VI Reference(vi path=w329, error in (no error)=w332) -> (vi reference=w333:refnum<vi>, error out=w334:errorcluster)  [unwired: 4 in]
        n146 = invoke class="VI" method="FP.Open"(reference=w333, error in=w334) -> (reference out=w336:refnum<vi>, error out=w337:errorcluster)  [unwired: 3 in, 3 out]
        n147 = Close Reference(reference=w336, error in (no error)=w337) -> (error out=w335:errorcluster)
        n148 = call <vilib>:"Simple Error Handler.vi"("error in (no error)"=w335) -> ("error out"=w331:errorcluster)  [unwired: 4 in, 4 out]
      }
      event "open_MCCETC01": Value Change {
        n149 = event-data() -> ()  [unwired: 1 in, 4 out]
        n150 = Index Array(array=w338, index=9) -> (element=w339:path)
        n151 = Open VI Reference(vi path=w339, error in (no error)=w342) -> (vi reference=w343:refnum<vi>, error out=w344:errorcluster)  [unwired: 4 in]
        n152 = invoke class="VI" method="FP.Open"(reference=w343, error in=w344) -> (reference out=w346:refnum<vi>, error out=w347:errorcluster)  [unwired: 3 in, 3 out]
        n153 = Close Reference(reference=w346, error in (no error)=w347) -> (error out=w345:errorcluster)
        n154 = call <vilib>:"Simple Error Handler.vi"("error in (no error)"=w345) -> ("error out"=w341:errorcluster)  [unwired: 4 in, 4 out]
      }
      event "open_MCCETC02": Value Change {
        n155 = event-data() -> ()  [unwired: 1 in, 4 out]
        n156 = Index Array(array=w349, index=10) -> (element=w348:path)
        n157 = Open VI Reference(vi path=w348, error in (no error)=w352) -> (vi reference=w353:refnum<vi>, error out=w354:errorcluster)  [unwired: 4 in]
        n158 = invoke class="VI" method="FP.Open"(reference=w353, error in=w354) -> (reference out=w356:refnum<vi>, error out=w357:errorcluster)  [unwired: 3 in, 3 out]
        n159 = Close Reference(reference=w356, error in (no error)=w357) -> (error out=w355:errorcluster)
        n160 = call <vilib>:"Simple Error Handler.vi"("error in (no error)"=w355) -> ("error out"=w351:errorcluster)  [unwired: 4 in, 4 out]
      }
      event "open_MCCETC03": Value Change {
        n161 = event-data() -> ()  [unwired: 1 in, 4 out]
        n162 = Index Array(array=w358, index=11) -> (element=w359:path)
        n163 = Open VI Reference(vi path=w359, error in (no error)=w362) -> (vi reference=w363:refnum<vi>, error out=w364:errorcluster)  [unwired: 4 in]
        n164 = invoke class="VI" method="FP.Open"(reference=w363, error in=w364) -> (reference out=w366:refnum<vi>, error out=w367:errorcluster)  [unwired: 3 in, 3 out]
        n165 = Close Reference(reference=w366, error in (no error)=w367) -> (error out=w365:errorcluster)
        n166 = call <vilib>:"Simple Error Handler.vi"("error in (no error)"=w365) -> ("error out"=w361:errorcluster)  [unwired: 4 in, 4 out]
      }
      event "open_LS218_01": Value Change {
        n167 = event-data() -> ()  [unwired: 1 in, 4 out]
        n168 = Index Array(array=w369, index=12) -> (element=w368:path)
        n169 = Open VI Reference(vi path=w368, error in (no error)=w372) -> (vi reference=w373:refnum<vi>, error out=w374:errorcluster)  [unwired: 4 in]
        n170 = invoke class="VI" method="FP.Open"(reference=w373, error in=w374) -> (reference out=w376:refnum<vi>, error out=w377:errorcluster)  [unwired: 3 in, 3 out]
        n171 = Close Reference(reference=w376, error in (no error)=w377) -> (error out=w375:errorcluster)
        n172 = call <vilib>:"Simple Error Handler.vi"("error in (no error)"=w375) -> ("error out"=w371:errorcluster)  [unwired: 4 in, 4 out]
      }
      event "open_LS218_02": Value Change {
        n173 = event-data() -> ()  [unwired: 1 in, 4 out]
        n174 = Index Array(array=w379, index=13) -> (element=w378:path)
        n175 = Open VI Reference(vi path=w378, error in (no error)=w382) -> (vi reference=w383:refnum<vi>, error out=w384:errorcluster)  [unwired: 4 in]
        n176 = invoke class="VI" method="FP.Open"(reference=w383, error in=w384) -> (reference out=w386:refnum<vi>, error out=w387:errorcluster)  [unwired: 3 in, 3 out]
        n177 = Close Reference(reference=w386, error in (no error)=w387) -> (error out=w385:errorcluster)
        n178 = call <vilib>:"Simple Error Handler.vi"("error in (no error)"=w385) -> ("error out"=w381:errorcluster)  [unwired: 4 in, 4 out]
      }
      event "open_LJU3_TC": Value Change {
        n179 = event-data() -> ()  [unwired: 1 in, 4 out]
        n180 = Index Array(array=w389, index=14) -> (element=w388:path)
        n181 = Open VI Reference(vi path=w388, error in (no error)=w392) -> (vi reference=w393:refnum<vi>, error out=w394:errorcluster)  [unwired: 4 in]
        n182 = invoke class="VI" method="FP.Open"(reference=w393, error in=w394) -> (reference out=w396:refnum<vi>, error out=w397:errorcluster)  [unwired: 3 in, 3 out]
        n183 = Close Reference(reference=w396, error in (no error)=w397) -> (error out=w395:errorcluster)
        n184 = call <vilib>:"Simple Error Handler.vi"("error in (no error)"=w395) -> ("error out"=w391:errorcluster)  [unwired: 4 in, 4 out]
      }
      event "open_LJT4": Value Change {
        n185 = event-data() -> ()  [unwired: 1 in, 4 out]
        n186 = Index Array(array=w400, index=15) -> (element=w399:path)
        n187 = Open VI Reference(vi path=w399, error in (no error)=w402) -> (vi reference=w403:refnum<vi>, error out=w404:errorcluster)  [unwired: 4 in]
        n188 = invoke class="VI" method="FP.Open"(reference=w403, error in=w404) -> (reference out=w406:refnum<vi>, error out=w407:errorcluster)  [unwired: 3 in, 3 out]
        n189 = Close Reference(reference=w406, error in (no error)=w407) -> (error out=w405:errorcluster)
        n190 = call <vilib>:"Simple Error Handler.vi"("error in (no error)"=w405) -> ("error out"=w401:errorcluster)  [unwired: 4 in, 4 out]
      }
      event "open_RPLCW": Value Change {
        n191 = event-data() -> ()  [unwired: 1 in, 4 out]
        n192 = Index Array(array=w409, index=16) -> (element=w408:path)
        n193 = Open VI Reference(vi path=w408, error in (no error)=w412) -> (vi reference=w413:refnum<vi>, error out=w414:errorcluster)  [unwired: 4 in]
        n194 = invoke class="VI" method="FP.Open"(reference=w413, error in=w414) -> (reference out=w416:refnum<vi>, error out=w417:errorcluster)  [unwired: 3 in, 3 out]
        n195 = Close Reference(reference=w416, error in (no error)=w417) -> (error out=w415:errorcluster)
        n196 = call <vilib>:"Simple Error Handler.vi"("error in (no error)"=w415) -> ("error out"=w411:errorcluster)  [unwired: 4 in, 4 out]
      }
      event "open_ITM10": Value Change {
        n197 = event-data() -> ()  [unwired: 1 in, 4 out]
        n198 = Index Array(array=w419, index=17) -> (element=w418:path)
        n199 = Open VI Reference(vi path=w418, error in (no error)=w422) -> (vi reference=w423:refnum<vi>, error out=w424:errorcluster)  [unwired: 4 in]
        n200 = invoke class="VI" method="FP.Open"(reference=w423, error in=w424) -> (reference out=w426:refnum<vi>, error out=w427:errorcluster)  [unwired: 3 in, 3 out]
        n201 = Close Reference(reference=w426, error in (no error)=w427) -> (error out=w425:errorcluster)
        n202 = call <vilib>:"Simple Error Handler.vi"("error in (no error)"=w425) -> ("error out"=w421:errorcluster)  [unwired: 4 in, 4 out]
      }
      event "open_MagPS": Value Change {
        n203 = event-data() -> ()  [unwired: 1 in, 4 out]
        n204 = Index Array(array=w429, index=18) -> (element=w428:path)
        n205 = Open VI Reference(vi path=w428, error in (no error)=w432) -> (vi reference=w433:refnum<vi>, error out=w434:errorcluster)  [unwired: 4 in]
        n206 = invoke class="VI" method="FP.Open"(reference=w433, error in=w434) -> (reference out=w436:refnum<vi>, error out=w437:errorcluster)  [unwired: 3 in, 3 out]
        n207 = Close Reference(reference=w436, error in (no error)=w437) -> (error out=w435:errorcluster)
        n208 = call <vilib>:"Simple Error Handler.vi"("error in (no error)"=w435) -> ("error out"=w431:errorcluster)  [unwired: 4 in, 4 out]
      }
      event "open_MRB": Value Change {
        n209 = event-data() -> ()  [unwired: 1 in, 4 out]
        n210 = Index Array(array=w438, index=19) -> (element=w439:path)
        n211 = Open VI Reference(vi path=w439, error in (no error)=w442) -> (vi reference=w443:refnum<vi>, error out=w444:errorcluster)  [unwired: 4 in]
        n212 = invoke class="VI" method="FP.Open"(reference=w443, error in=w444) -> (reference out=w446:refnum<vi>, error out=w447:errorcluster)  [unwired: 3 in, 3 out]
        n213 = Close Reference(reference=w446, error in (no error)=w447) -> (error out=w445:errorcluster)
        n214 = call <vilib>:"Simple Error Handler.vi"("error in (no error)"=w445) -> ("error out"=w441:errorcluster)  [unwired: 4 in, 4 out]
      }
      event "open_GVB": Value Change {
        n215 = event-data() -> ()  [unwired: 1 in, 4 out]
        n216 = Index Array(array=w449, index=20) -> (element=w448:path)
        n217 = Open VI Reference(vi path=w448, error in (no error)=w452) -> (vi reference=w453:refnum<vi>, error out=w454:errorcluster)  [unwired: 4 in]
        n218 = invoke class="VI" method="FP.Open"(reference=w453, error in=w454) -> (reference out=w456:refnum<vi>, error out=w457:errorcluster)  [unwired: 3 in, 3 out]
        n219 = Close Reference(reference=w456, error in (no error)=w457) -> (error out=w455:errorcluster)
        n220 = call <vilib>:"Simple Error Handler.vi"("error in (no error)"=w455) -> ("error out"=w451:errorcluster)  [unwired: 4 in, 4 out]
      }
      event "open_MccHat": Value Change {
        n221 = event-data() -> ()  [unwired: 1 in, 4 out]
        n222 = Index Array(array=w459, index=21) -> (element=w458:path)
        n223 = Open VI Reference(vi path=w458, error in (no error)=w462) -> (vi reference=w463:refnum<vi>, error out=w464:errorcluster)  [unwired: 4 in]
        n224 = invoke class="VI" method="FP.Open"(reference=w463, error in=w464) -> (reference out=w466:refnum<vi>, error out=w467:errorcluster)  [unwired: 3 in, 3 out]
        n225 = Close Reference(reference=w466, error in (no error)=w467) -> (error out=w465:errorcluster)
        n226 = call <vilib>:"Simple Error Handler.vi"("error in (no error)"=w465) -> ("error out"=w461:errorcluster)  [unwired: 4 in, 4 out]
      }
      event "open_Heat_Tape": Value Change {
        n227 = event-data() -> ()  [unwired: 1 in, 4 out]
        n228 = Index Array(array=w469, index=22) -> (element=w468:path)
        n229 = Open VI Reference(vi path=w468, error in (no error)=w472) -> (vi reference=w473:refnum<vi>, error out=w474:errorcluster)  [unwired: 4 in]
        n230 = invoke class="VI" method="FP.Open"(reference=w473, error in=w474) -> (reference out=w476:refnum<vi>, error out=w477:errorcluster)  [unwired: 3 in, 3 out]
        n231 = Close Reference(reference=w476, error in (no error)=w477) -> (error out=w475:errorcluster)
        n232 = call <vilib>:"Simple Error Handler.vi"("error in (no error)"=w475) -> ("error out"=w471:errorcluster)  [unwired: 4 in, 4 out]
      }
      event "open_IVC_OC200": Value Change {
        n233 = event-data() -> ()  [unwired: 1 in, 4 out]
        n234 = Index Array(array=w479, index=23) -> (element=w478:path)
        n235 = Open VI Reference(vi path=w478, error in (no error)=w482) -> (vi reference=w483:refnum<vi>, error out=w484:errorcluster)  [unwired: 4 in]
        n236 = invoke class="VI" method="FP.Open"(reference=w483, error in=w484) -> (reference out=w486:refnum<vi>, error out=w487:errorcluster)  [unwired: 3 in, 3 out]
        n237 = Close Reference(reference=w486, error in (no error)=w487) -> (error out=w485:errorcluster)
        n238 = call <vilib>:"Simple Error Handler.vi"("error in (no error)"=w485) -> ("error out"=w481:errorcluster)  [unwired: 4 in, 4 out]
      }
    }
  }
  n239 = property on="stop" class="Bool (strict)"(error in=w2, "Value"=FALSE ("stop")) -> ()  [unwired: 1 in, 2 out]
